vi "TPNT_CleanAllData.vi"(8 "error in (no error)":errorcluster) -> (0 "error out":errorcluster)   [LabVIEW 2016]
uses:
  TPNT_CoreFunction.ctl
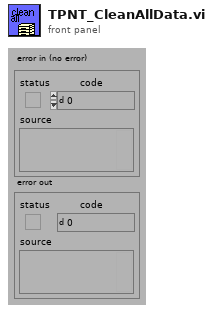
[diagram p1: front panel]
types:
  T1 = typedef "TPNT_CoreFunction.ctl" = enum16{"Reset", "Register", "Get Data", "Set Data", "Unregister", "Test", "Get Objects"}
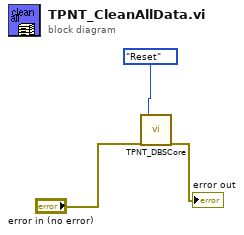
[diagram p0: block diagram]
diagram:
  n1 = call "TPNT_DBSCore.vi"("error in (no error)"="error in (no error)", "Function (Get Data)"=TPNT_CoreFunction."Reset") -> ("error out"=→"error out":errorcluster)  [unwired: 3 in, 14 out]
